vi "Ev Frame Num.vi"(8 "error in (no error)":errorcluster, 10 "Old Value":u32, 11 "IDE simple in":refnum<class "Main Panel.lvclass">) -> (0 "error out":errorcluster, 3 "IDE simple out":refnum<class "Main Panel.lvclass">)   [LabVIEW 2018, in "Main Panel.lvlib" / "Main Panel.lvclass"]
uses:
  Main Panel.lvclass
  Main Panel.lvclass/Main Panel.ctl
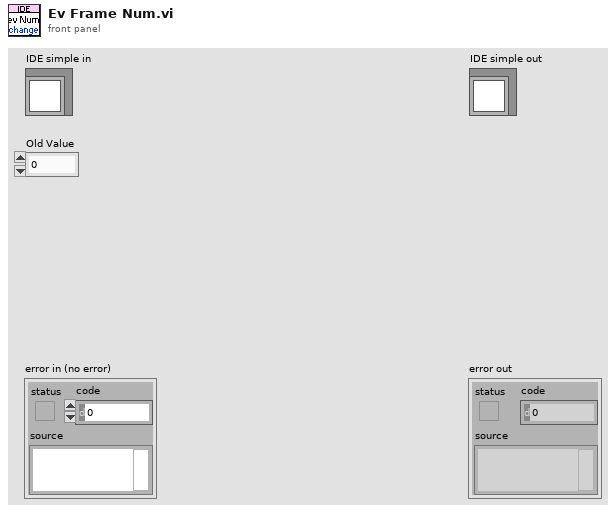
[diagram p1: front panel]
types:
  T1 = enum16{"Left Button", "Center Button", "Right Button", "Window Close"}
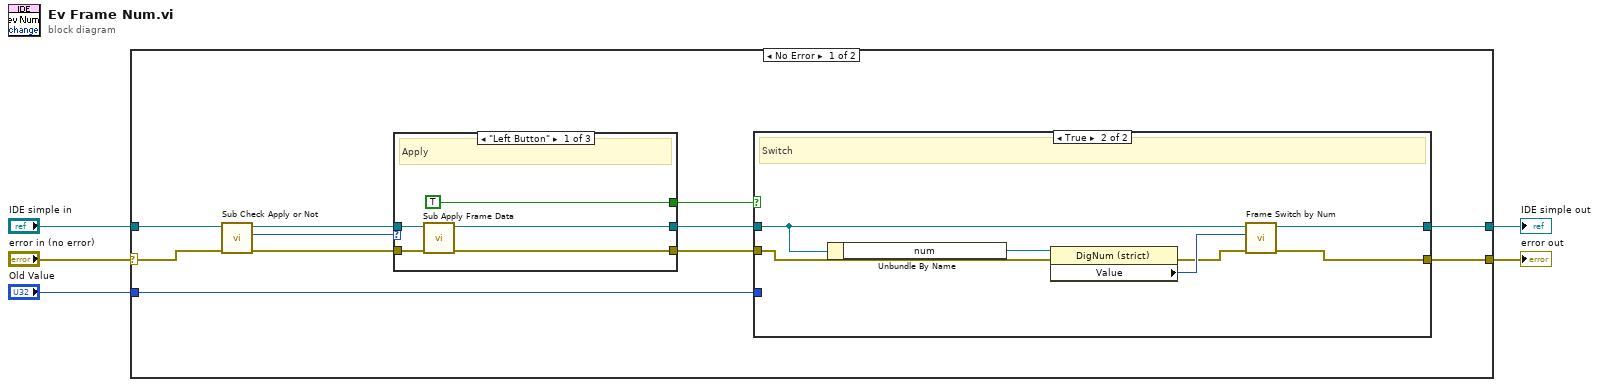
[diagram p0: block diagram]
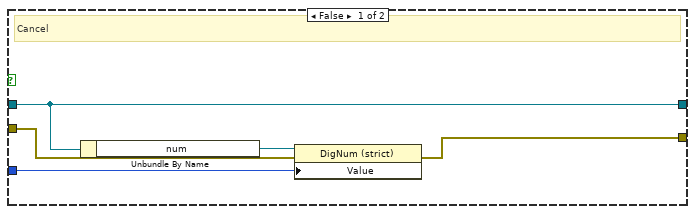
[diagram p2: hidden frame]
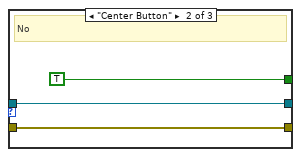
[diagram p3: hidden frame]
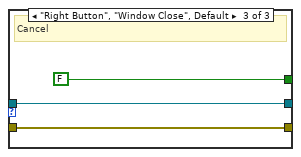
[diagram p4: hidden frame]
diagram:
  n1 = case shown="No Error" "error in (no error)" {
    selector: "error in (no error)" -> [w9 w40]
    tunnel: [w14 w40] -> w4
    tunnel: [w15 w39] -> w2
    tunnel: "IDE simple in" -> [w10 w39]
    tunnel: "Old Value" -> [w6 _]
    frame No Error {
      n2 = call "Sub Check Apply or Not.vi"("error in (no error)"=w9, "Main Panel in"=w10) -> ("error out"=w11:errorcluster, "Which Button?"=w13:T1, "Main Panel out"=w12:refnum<class "Main Panel.lvclass">)  [unwired: 7 in]
      n3 = case shown="\"Left Button\"" w13 {
        tunnel: w12 -> [w32 w35 w38]
        tunnel: w11 -> [w31 w34 w37]
        tunnel: [w30 w35 w38] -> _
        tunnel: [w29 w34 w37] -> w8
        tunnel: [TRUE TRUE FALSE] -> w7
        frame "Left Button" {
          # "Apply"
          n4 = call "Sub Apply Frame Data.vi"("error in (no error)"=w31, "IDE simple in"=w32) -> ("error out"=w29:errorcluster, "IDE simple out"=w30:refnum<class "Main Panel.lvclass">)  [unwired: 8 in]
        }
        frame "Center Button" {
          # "No"
        }
        frame "Right Button", "Window Close", Default {
          # "Cancel"
        }
      }
      n5 = case shown="True" w7 {
        tunnel: [w16 w24] -> w15
        tunnel: [w17 w23] -> w14
        tunnel: w10 -> [w16 w22]
        tunnel: w8 -> [w18 w21]
        tunnel: w6 -> [w19 _]
        frame False {
          # "Cancel"
          n6 = Unbundle By Name(w16) -> ("num"=w20:refnum<vi>)
          n7 = property class="DigNum (strict)"(reference=w20, error in=w18, "Value"=w19) -> (error out=w17:errorcluster)  [unwired: 1 out]
        }
        frame True {
          # "Switch"
          n8 = Unbundle By Name(w22) -> ("num"=w27:refnum<vi>)
          n9 = property class="DigNum (strict)"(reference=w27, error in=w21) -> (error out=w25:errorcluster, "Value"=w26:u32)  [unwired: 1 out]
          n10 = call "Frame Switch by Num.vi"("error in (no error)"=w25, "Frame Num"=w26, "LF2R IDE in"=w22) -> ("error out"=w23:errorcluster, "LF2R IDE out"=w24:refnum<class "Main Panel.lvclass">)  [unwired: 7 in]
        }
      }
    }
    frame Error {
    }
  }
  "error out" <- w4
  "IDE simple out" <- w2
